vi "RTT_Sample_App.vi"() -> ()   [LabVIEW 2011]
uses:
  Lib/JLinkARM.lvlib
panel:
  out "Read loop done":bool
  out "Write loop done":bool
  in  "RTT - Host -> Target 2":string
  in  "Send RTT Data":bool
  out "Num bytes read total":u32
  out "RTT - Target -> Host":string
  out "Error":bool
  out "RTT active":bool
  out "Connect successful":bool
  out "Output":string
  in  "Use IP":bool
  in  "IP:":string
  in  "STOP RTT":bool
  in  "Serial Number:":dbl
  in  "Interface:":i32(listbox)
  in  "TIF Speed [kHz]:":dbl
  in  "Device:":string
  in  "START RTT":bool
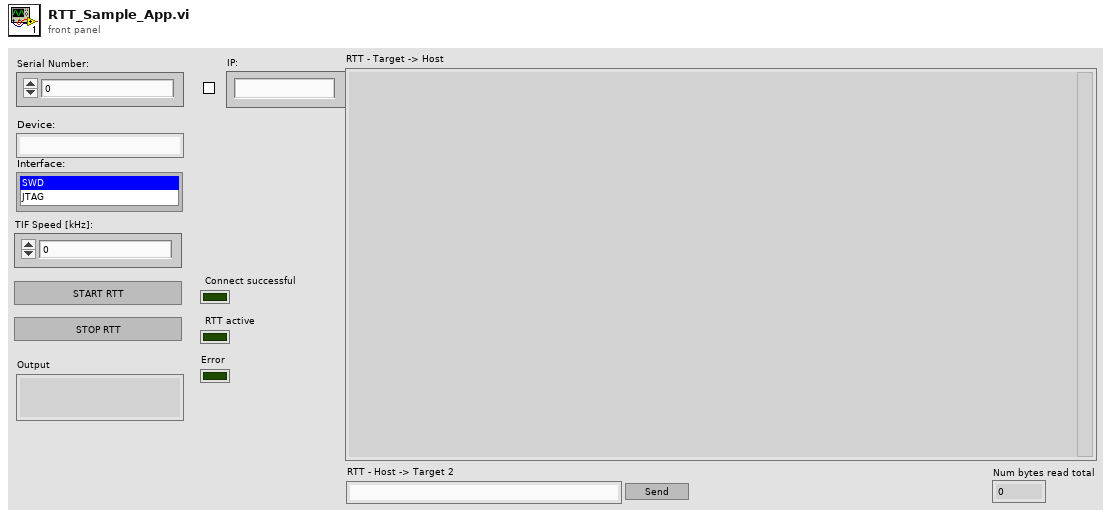
[diagram p1: front panel]
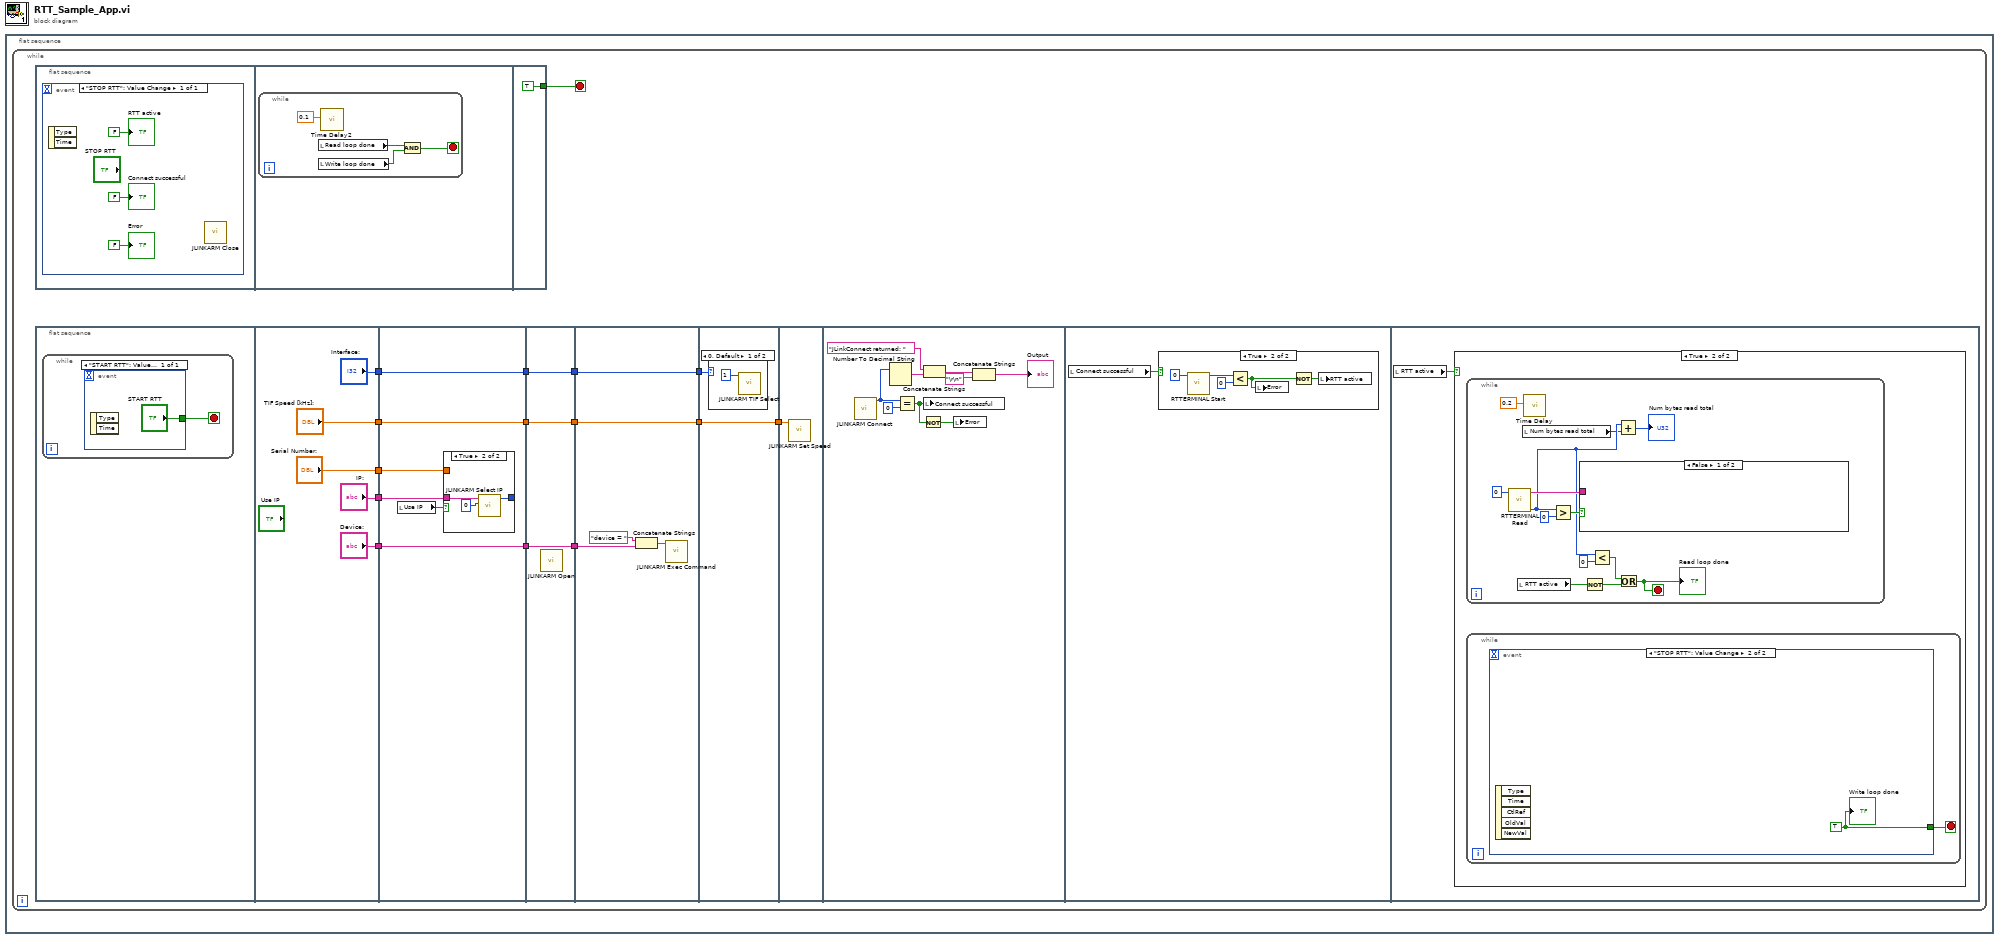
[diagram p0: block diagram]
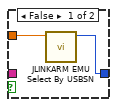
[diagram p2: hidden frame]
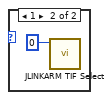
[diagram p3: hidden frame]
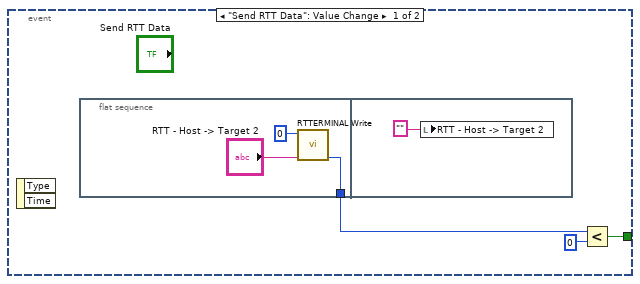
[diagram p6: hidden frame]
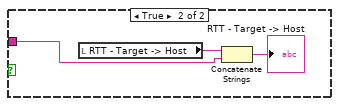
[diagram p7: hidden frame]
diagram:
  n1 = flat-sequence {
    frame #0 {
      n2 = while {
        stop <- w1 stop-if-true
        n3 = flat-sequence {
          tunnel: [TRUE] -> w1
          frame #0 {
            n4 = event shown="[0] \"STOP RTT\": Value Change" {
              selector: _ -> [_]
              dyn-events: _ -> [_]
              timeout: _ -> [_]
              event "STOP RTT": Value Change {
                n5 = event-data() -> ()  [unwired: 1 in, 2 out]
                n6 = call "JLINKARM Close.vi"() -> ()  [unwired: 12 in]
                "RTT active" <- FALSE
                "Connect successful" <- FALSE
                "Error" <- FALSE
              }
            }
          }
          frame #1 {
            n7 = while {
              stop <- w20 stop-if-true
              n8 = local read "Read loop done"() -> (w22:bool)
              n9 = local read "Write loop done"() -> (w21:bool)
              n10 = call "Time Delay2"("Delay Time (s)"=0.1) -> ()  [unwired: 10 in, 1 out]
              n11 = And(x=w22, y=w21) -> (x .and. y?=w20:bool)
            }
          }
          frame #2 {
          }
        }
        n12 = flat-sequence {
          tunnel: ["Serial Number:"] -> w15
          tunnel: ["Interface:"] -> w11
          tunnel: ["TIF Speed [kHz]:"] -> w10
          tunnel: ["Device:"] -> w3
          tunnel: ["IP:"] -> w2
          tunnel: w15 -> [w32]
          tunnel: [w36] -> w12
          tunnel: w11 -> [w36]
          tunnel: w10 -> [w35]
          tunnel: [w35] -> w9
          tunnel: [w34] -> w4
          tunnel: w3 -> [w34]
          tunnel: w2 -> [w33]
          tunnel: [w44] -> w13
          tunnel: w12 -> [w44]
          tunnel: w9 -> [w43]
          tunnel: [w43] -> w8
          tunnel: [w42] -> w5
          tunnel: w4 -> [w42]
          tunnel: [w49] -> w14
          tunnel: w13 -> [w49]
          tunnel: w8 -> [w48]
          tunnel: [w48] -> w7
          tunnel: w5 -> [w46]
          tunnel: w14 -> [w51]
          tunnel: w7 -> [w50]
          tunnel: [w50] -> w6
          tunnel: w6 -> [w54]
          frame #0 {
            n13 = while {
              stop <- w24 stop-if-true
              n14 = event shown="[0] \"START RTT\": Value Change" {
                selector: _ -> [_]
                dyn-events: _ -> [_]
                timeout: _ -> [_]
                tunnel: ["START RTT"] -> w24
                event "START RTT": Value Change {
                  n15 = event-data() -> ()  [unwired: 1 in, 2 out]
                }
              }
            }
          }
          frame #1 {
          }
          frame #2 {
            n16 = local read "Use IP"() -> (w31:bool)
            n17 = case shown="True" w31 {
              tunnel: w33 -> [_ w41]
              tunnel: w32 -> [w38 _]
              tunnel: [w37 w39] -> _
              frame False {
                n18 = call "JLINKARM EMU Select By USBSN.vi"("SerialNo"=w38) -> ("function return"=w37:i32)  [unwired: 10 in]
              }
              frame True {
                n19 = call "JLINKARM Select IP.vi"("Port"=0, "sHost"=w41) -> ("function return"=w39:i8)  [unwired: 9 in]
              }
            }
          }
          frame #3 {
            n20 = call "JLINKARM Open.vi"() -> ()  [unwired: 11 in, 1 out]
          }
          frame #4 {
            n21 = Concatenate Strings("device = ", w46) -> (w45:string)
            n22 = call "JLINKARM Exec Command.vi"("pIn"=w45) -> ()  [unwired: 9 in, 2 out]
          }
          frame #5 {
            n23 = case shown="0, Default" w51 {
              frame 0, Default {
                n24 = call "JLINKARM TIF Select.vi"("Interface"=1) -> ()  [unwired: 10 in, 1 out]
              }
              frame 1 {
                n25 = call "JLINKARM TIF Select.vi"("Interface"=0) -> ()  [unwired: 10 in, 1 out]
              }
            }
          }
          frame #6 {
            n26 = call "JLINKARM Set Speed.vi"("Speed"=w54) -> ()  [unwired: 11 in]
          }
          frame #7 {
            n27 = call "JLINKARM Connect.vi"() -> ("function return"=w58:i32)  [unwired: 11 in]
            n28 = Number To Decimal String(number=w58) -> (decimal integer string=w60:string)  [unwired: 1 in]
            n29 = Equal?(x=w58, y=0) -> (x = y?=w56:bool)
            n30 = Not(x=w56) -> (.not. x?=w55:bool)
            n31 = Concatenate Strings("JLinkConnect returned: ", w60) -> (w57:string)
            n32 = local write "Connect successful"(w56) -> ()
            n33 = local write "Error"(w55) -> ()
            n34 = Concatenate Strings(w57, "\r\n") -> (→"Output":string)
          }
          frame #8 {
            n35 = local read "Connect successful"() -> (w64:bool)
            n36 = case shown="True" w64 {
              frame False {
              }
              frame True {
                n37 = call "RTTERMINAL Start.vi"("Control block address [hex]"=0) -> ("function return"=w67:i32)  [unwired: 10 in]
                n38 = Less?(x=w67, y=0) -> (x < y?=w65:bool)
                n39 = local write "Error"(w65) -> ()
                n40 = Not(x=w65) -> (.not. x?=w69:bool)
                n41 = local write "RTT active"(w69) -> ()
              }
            }
          }
          frame #9 {
            n42 = local read "RTT active"() -> (w70:bool)
            n43 = case shown="True" w70 {
              frame False {
              }
              frame True {
                n44 = while {
                  stop <- w80 stop-if-true
                  n45 = call "RTTERMINAL Read.vi"("BufferIndex"=0) -> ("Return"=w86:i32, "Data from target"=w88:string)  [unwired: 9 in]
                  n46 = local read "RTT active"() -> (w81:bool)
                  n47 = local read "Num bytes read total"() -> (w85:u32)
                  n48 = call "Time Delay"("Delay Time (s)"=0.2) -> ()  [unwired: 10 in, 1 out]
                  n49 = Greater?(x=w86, y=0) -> (0:w87:bool)
                  n50 = case shown="False" w87 {
                    tunnel: w88 -> [_ w95]
                    frame False {
                    }
                    frame True {
                      n51 = local read "RTT - Target -> Host"() -> (w93:string)
                      n52 = Concatenate Strings(w93, w95) -> (→"RTT - Target -> Host":string)
                    }
                  }
                  n53 = Not(x=w81) -> (.not. x?=w82:bool)
                  n54 = Less?(x=w86, y=0) -> (x < y?=w83:bool)
                  n55 = Add(x=w86, y=w85) -> (x+y=→"Num bytes read total":u32)
                  n56 = Or(x=w83, y=w82) -> (x .or. y?=w80:bool)
                  "Read loop done" <- w80
                }
                n57 = while {
                  stop <- w71 stop-if-true
                  n58 = event shown="[1] \"STOP RTT\": Value Change" {
                    selector: _ -> [_ _]
                    dyn-events: _ -> [_ _]
                    timeout: _ -> [_ _]
                    tunnel: [w72 w79] -> w71
                    event "Send RTT Data": Value Change {
                      n59 = event-data() -> ()  [unwired: 1 in, 2 out]
                      n60 = flat-sequence {
                        tunnel: [w75] -> w74
                        frame #0 {
                          n61 = call "RTTERMINAL Write.vi"("RTT Write"="RTT - Host -> Target 2", "Down buffer index"=0) -> ("Return"=w75:i32)  [unwired: 9 in]
                        }
                        frame #1 {
                          n62 = local write "RTT - Host -> Target 2"("" ("RTT - Host -> Target 2")) -> ()
                        }
                      }
                      n63 = Less?(x=w74, y=0) -> (x < y?=w72:bool)
                    }
                    event "STOP RTT": Value Change {
                      w79 = TRUE
                      n64 = event-data() -> ()  [unwired: 1 in, 5 out]
                      "Write loop done" <- w79
                    }
                  }
                }
              }
            }
          }
        }
      }
    }
  }
